vi "Limit Switch Control.vi"(11 "Run Mode":T1) -> (0 "Limit Switch 4":bool, 1 "Limit Switch 3":bool, 2 "Limit Switch 2":bool, 3 "Limit Switch 1":bool)   [LabVIEW 2014]
uses:
  Controls/SRE Enum.ctl
  Text Variable VIs/Read Number Variable.vi
  <vilib>/Rock Robotics/WPI/Switch/WPI_SwitchOpenLimit.vi
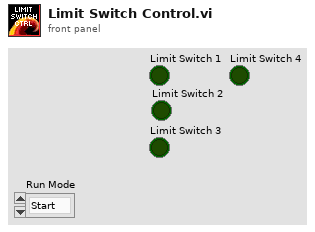
[diagram p1: front panel]
types:
  T1 = typedef "SRE Enum.ctl" = enum16{"Start", "Run", "End"}
  T2 = typedef "WPI_SwitchDevRef.ctl" = cluster{"DevStatus":errorcluster, "DIO Channel":T3, "Controller":T4, "CntIndex":T5, "Normally Closed":bool}
  T3 = typedef "FPGA_DIOChannel.ctl" = enum8{"DIO 0", "DIO 1", "DIO 2", "DIO 3", "DIO 4", "DIO 5", "DIO 6", "DIO 7", "DIO 8", "DIO 9", "DIO MXP 0", "DIO MXP 1", "DIO MXP 2", "DIO MXP 3", "DIO MXP 4", "DIO MXP 5", "DIO MXP 6", "DIO MXP 7", "DIO MXP 8", "DIO MXP 9", "DIO MXP 10", "DIO MXP 11", "DIO MXP 12", "DIO MXP 13", "DIO MXP 14", "DIO MXP 15", "Invalid"}
  T4 = typedef "FPGA_TypedefDigitalModule.ctl" = enum16{"Controller 1"}
  T5 = typedef "FPGA_CounterCtrSystemIndex.ctl" = enum8{"Ctr 0", "Ctr 1", "Ctr 2", "Ctr 3", "Ctr 4", "Ctr 5", "Ctr 6", "Ctr 7", "Invalid"}
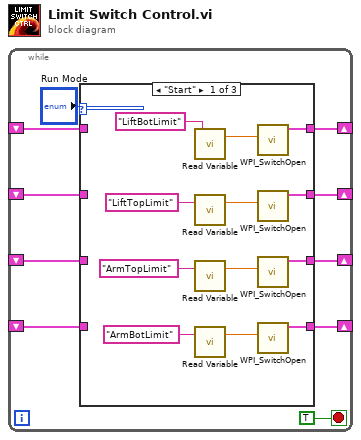
[diagram p0: block diagram]
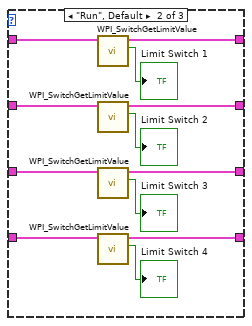
[diagram p2: hidden frame]
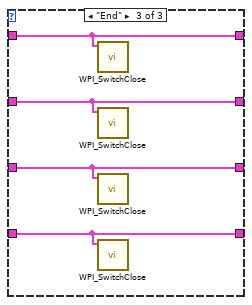
[diagram p3: hidden frame]
diagram:
  n1 = while {
    shift-right: [w7] -> _
    shift-left: _ -> [w4]
    shift-right: [w8] -> _
    shift-left: _ -> [w5]
    shift-right: [w9] -> _
    shift-left: _ -> [w3]
    shift-right: [w6] -> _
    shift-left: _ -> [w2]
    stop <- TRUE stop-if-true
    n2 = case shown="\"Start\"" "Run Mode" {
      tunnel: [w22 w30 w37] -> w9
      tunnel: [w21 w31 w36] -> w8
      tunnel: [w20 w33 w35] -> w7
      tunnel: [w19 w27 w38] -> w6
      tunnel: w5 -> [_ w32 w36]
      tunnel: w4 -> [_ w34 w35]
      tunnel: w3 -> [_ w29 w37]
      tunnel: w2 -> [_ w28 w38]
      frame "Start" {
        n3 = call-poly "Read Variable.vi"("Name"="LiftBotLimit") -> ("number"=w15:dbl)  [unwired: 1 in, 1 out]
        n4 = call-poly "Read Variable.vi"("Name"="LiftTopLimit") -> ("number"=w16:dbl)  [unwired: 1 in, 1 out]
        n5 = call-poly "Read Variable.vi"("Name"="ArmTopLimit") -> ("number"=w17:dbl)  [unwired: 1 in, 1 out]
        n6 = call-poly "Read Variable.vi"("Name"="ArmBotLimit") -> ("number"=w18:dbl)  [unwired: 1 in, 1 out]
        n7 = call-poly <vilib>:"WPI_SwitchOpen.vi"("DIO Channel"=w15) -> ("SwitchDevRef"=w20:T2)  [unwired: 9 in, 1 out]
        n8 = call-poly <vilib>:"WPI_SwitchOpen.vi"("DIO Channel"=w16) -> ("SwitchDevRef"=w21:T2)  [unwired: 9 in, 1 out]
        n9 = call-poly <vilib>:"WPI_SwitchOpen.vi"("DIO Channel"=w17) -> ("SwitchDevRef"=w22:T2)  [unwired: 9 in, 1 out]
        n10 = call-poly <vilib>:"WPI_SwitchOpen.vi"("DIO Channel"=w18) -> ("SwitchDevRef"=w19:T2)  [unwired: 9 in, 1 out]
      }
      frame "Run", Default {
        n11 = call <vilib>:"WPI_SwitchGetLimitValue.vi"("SwitchDevRef"=w34) -> ("Switch Pressed"=→"Limit Switch 1":bool, "SwitchDevRef"=w33:T2)  [unwired: 8 in, 1 out]
        n12 = call <vilib>:"WPI_SwitchGetLimitValue.vi"("SwitchDevRef"=w32) -> ("Switch Pressed"=→"Limit Switch 2":bool, "SwitchDevRef"=w31:T2)  [unwired: 8 in, 1 out]
        n13 = call <vilib>:"WPI_SwitchGetLimitValue.vi"("SwitchDevRef"=w29) -> ("Switch Pressed"=→"Limit Switch 3":bool, "SwitchDevRef"=w30:T2)  [unwired: 8 in, 1 out]
        n14 = call <vilib>:"WPI_SwitchGetLimitValue.vi"("SwitchDevRef"=w28) -> ("Switch Pressed"=→"Limit Switch 4":bool, "SwitchDevRef"=w27:T2)  [unwired: 8 in, 1 out]
      }
      frame "End" {
        n15 = call <vilib>:"WPI_SwitchClose.vi"("SwitchDevRef"=w35) -> ()  [unwired: 10 in, 1 out]
        n16 = call <vilib>:"WPI_SwitchClose.vi"("SwitchDevRef"=w36) -> ()  [unwired: 10 in, 1 out]
        n17 = call <vilib>:"WPI_SwitchClose.vi"("SwitchDevRef"=w37) -> ()  [unwired: 10 in, 1 out]
        n18 = call <vilib>:"WPI_SwitchClose.vi"("SwitchDevRef"=w38) -> ()  [unwired: 10 in, 1 out]
      }
    }
  }
